vi "set.vi"(8 "error in (no error)":errorcluster caption="错误输入（无错误）", 10 "Url":string, 11 "HttpClient输入":refnum<class "Http.lvclass">) -> (0 "error out":errorcluster caption="错误输出", 3 "HttpClient输出":refnum<class "Http.lvclass">)   [LabVIEW 2012, in "Http.lvclass"]
uses:
  Http.lvclass
  Http.lvclass/Http.ctl
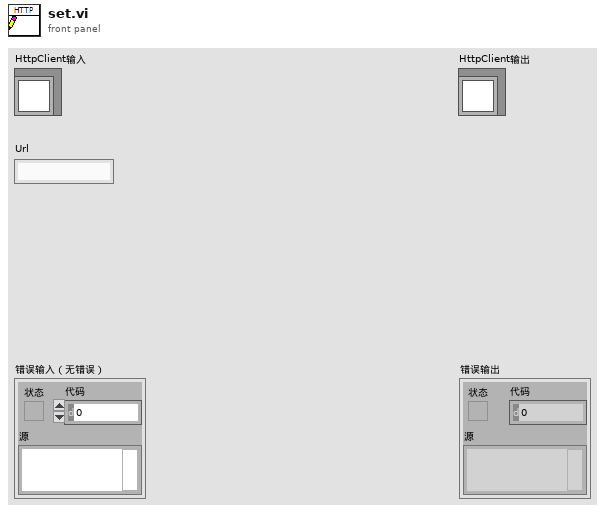
[diagram p1: front panel]
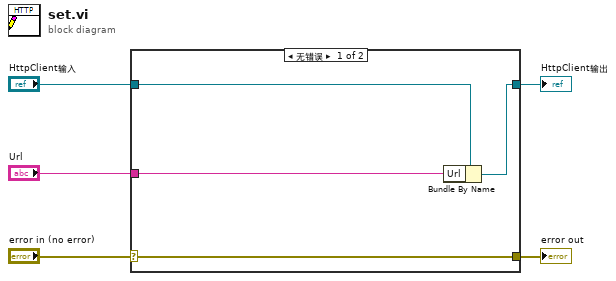
[diagram p0: block diagram]
diagram:
  n1 = case shown="无错误" "error in (no error)" {
    selector: "error in (no error)" -> [w9 w10]
    tunnel: [w9 w10] -> w4
    tunnel: [w7 w11] -> w2
    tunnel: "HttpClient输入" -> [w8 w11]
    tunnel: "Url" -> [w6 _]
    frame No Error {
      n2 = Bundle By Name(cluster=w8, "Url"=w6) -> (w7:refnum<class "Http.lvclass">)
    }
    frame Error {
    }
  }
  "error out" <- w4
  "HttpClient输出" <- w2
